vi "get Pol.vi"(10 "pol":i32, 11 "devID":u32) -> (2 "pol out":i32, 3 "function return":i32)   [LabVIEW 2014, in "libchaos-driver-powersupply-labview.lvlib"]
doc: "int getPol(unsigned int devID,int*pol);"
uses:
  libchaos-driver-powersupply-labview.lvlib
  chaos-i686-dynamic-release/lib/libchaos-driver-powersupply-labview.so
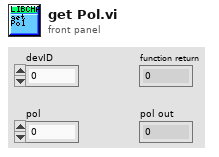
[diagram p1: front panel]
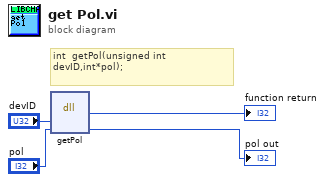
[diagram p0: block diagram]
diagram:
  # "int  getPol(unsigned int devID,int*pol);"
  n1 = dll-call lib="home/chaos/chaos_bundle/chaos-i686-dynamic-release/lib/libchaos-driver-powersupply-labview.*" fn="getPol"("devID"="devID", "pol"="pol") -> (→"function return":i32, "pol"=→"pol out":i32)  [unwired: 4 in, 2 out]
